vi "Configure Sweep Scan Signal.vi"(6 "Scan Dwelling (2 s)":dbl=2.0, 7 "Scan Steps (10)":u32=10, 8 "error in (no error)":errorcluster, 9 "Scan Amplitude (30 V)":dbl=30.0, 10 "Wait? (Off)":bool, 11 "VISA resource name":refnum<visa-resource-name>) -> (0 "error out":errorcluster, 3 "VISA resource name out":refnum<visa-resource-name>)   [LabVIEW 2017, in "DmmPwr Simulator.lvlib"]
doc: "Configures the amplitude and position for the scan signal."
uses:
  DmmPwr Simulator.lvlib
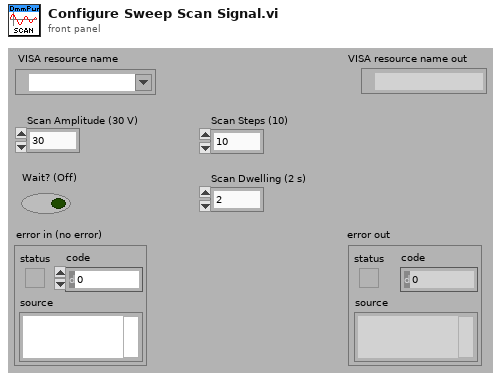
[diagram p1: front panel]
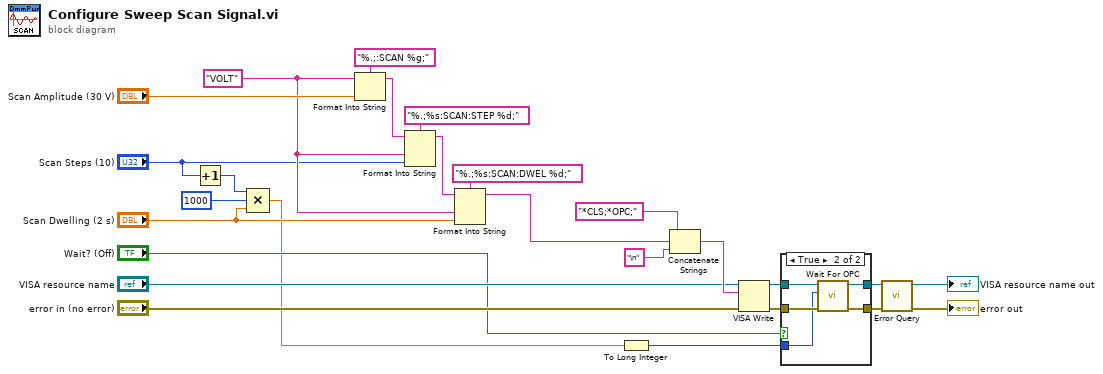
[diagram p0: block diagram]
diagram:
  w18 = "VOLT"
  n1 = Increment(x="Scan Steps (10)") -> (x+1=w3:u32)
  n2 = Compound Arithmetic op=MULTIPLY(w3, u32 1000 ("value"), "Scan Dwelling (2 s)") -> (w2:dbl)
  n3 = Format Into String(format string="%.;:SCAN %g;", initial string=w18, "Scan Amplitude (30 V)") -> (resulting string=w24:string)  [unwired: 1 in, 1 out]
  n4 = Format Into String(format string="%.;%s:SCAN:STEP %d;", initial string=w24, w18, "Scan Steps (10)") -> (resulting string=w22:string)  [unwired: 1 in, 1 out]
  n5 = Format Into String(format string="%.;%s:SCAN:DWEL %d;", initial string=w22, w18, "Scan Dwelling (2 s)") -> (resulting string=w14:string)  [unwired: 1 in, 1 out]
  n6 = To Long Integer(number=w2) -> (32bit integer=w1:i32)
  n7 = Concatenate Strings("*CLS;*OPC;" ("string"), w14, "\n" ("string")) -> (w17:string)
  n8 = VISA Write(VISA resource name="VISA resource name", write buffer=w17, error in (no error)="error in (no error)") -> (VISA resource name out=w12:refnum<visa-resource-name>, error out=w9:errorcluster)  [unwired: 1 out]
  n9 = case shown="True" "Wait? (Off)" {
    tunnel: w12 -> [w28 w33]
    tunnel: [w28 w32] -> w11
    tunnel: [w27 w31] -> w10
    tunnel: w9 -> [w27 w30]
    tunnel: w1 -> [_ w29]
    frame False {
    }
    frame True {
      n10 = call "Wait For OPC.vi"("error in"=w30, "Timeout (10000 ms)"=w29, "VISA resource name"=w33) -> ("error out"=w31:errorcluster, "VISA resource name out"=w32:refnum<visa-resource-name>)  [unwired: 7 in]
    }
  }
  n11 = call "Error Query.vi"("error in (no error)"=w10, "VISA resource name"=w11) -> ("error out"=→"error out":errorcluster, "VISA resource name out"=→"VISA resource name out":refnum<visa-resource-name>)  [unwired: 6 in, 2 out]
